vi "SetRegister_Sylap.vi"(8 "error in (no error)":errorcluster, 9 "Input Value":u64 format="%x", 10 "Register Name":u16(ring) items=["Enable"=0, "TotalOffsetCoarse"=1, "PulseLength"=2, "LaserHalfLength"=3, "LaserMaxCount"=4, "TotalOffset"=17, "ResetCounters"=18, "Reset"=16], 11 "VISA resource name":refnum<visa-resource-name>) -> (0 "error out":errorcluster, 1 "appended array":u32[](array[numeric]) format="%x", 2 "string":string, 3 "VISA resource name out":refnum<visa-resource-name>)   [LabVIEW 2020]
panel:
  out "Input Value 2":u64
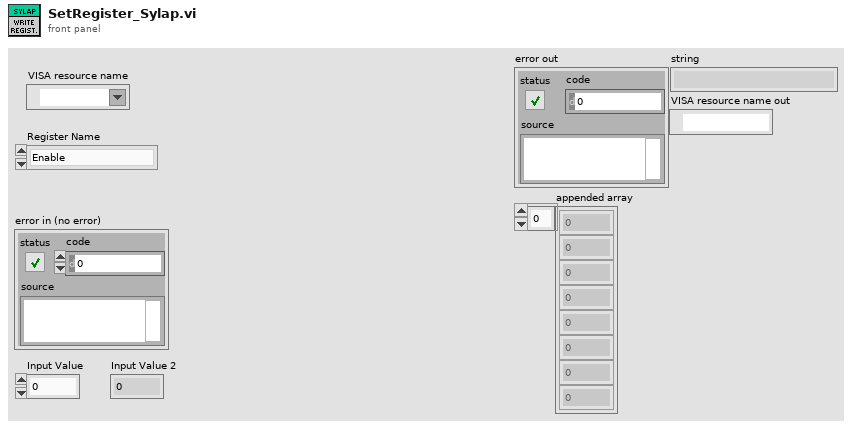
[diagram p1: front panel]
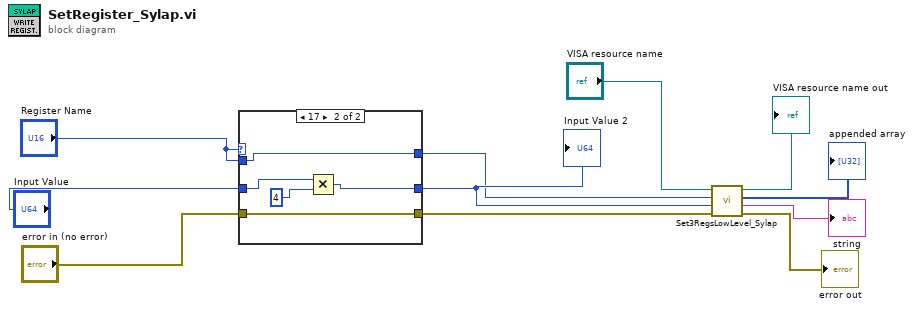
[diagram p0: block diagram]
diagram:
  n1 = case shown="17" "Register Name" {
    tunnel: "Register Name" -> [w12 w19]
    tunnel: "error in (no error)" -> [w14 w18]
    tunnel: [w12 w19] -> w7
    tunnel: [w14 w18] -> w10
    tunnel: "Input Value" -> [w13 w16]
    tunnel: [w13 w15] -> w8
    frame 0, Default {
    }
    frame 17 {
      n2 = Multiply(x=w16, y=4) -> (x*y=w15:u64)
    }
  }
  "Input Value 2" <- w8
  n3 = call "Set3RegsLowLevel_Sylap.vi"("error in (no error)"=w10, "Input Value"=w8, "Reg"=w7, "VISA resource name"="VISA resource name") -> ("error out"=→"error out":errorcluster, "string"=→"string":string, "appended array"=→"appended array":u32[], "VISA resource name out"=→"VISA resource name out":refnum<visa-resource-name>)  [unwired: 4 in]
